vi "断电保存变量.vi"() -> ()   [LabVIEW 2016, in "斯坦道多参数.lvlib"]
panel:
  in  "盐度自动获取":bool=TRUE
  out "大气压补偿":dbl=101.35
  out "盐度补偿":dbl
  in  "浊度标液2":dbl
  in  "浊度标液1":dbl
  in  "DO标液2":dbl
  in  "DO标液1":dbl
  in  "叶绿素a标液2":dbl
  in  "叶绿素a标液1":dbl
  in  "pH温度偏移补偿":dbl
  in  "Turb温度偏移补偿":dbl
  in  "Cond温度偏移补偿":dbl
  in  "DO温度偏移补偿":dbl
  in  "水样测定时间":dbl=1.0
  in  "叶绿素a启用":bool
  in  "标样核查配置":T1={"数据保存间隔"=1.0, "水温标样值"=0.0, "pH标样值"=0.0, "溶解氧标样值"=0.0, "电导率标样值"=0.0, "浊度标样值"=0.0}
  in  "Temp":bool
  in  "Cond":bool
  in  "Turb":bool
  in  "DO":bool
  in  "pH":bool
  in  "VISA资源名称":refnum<visa-resource-name>
  in  "水温通道":enum16{"NULL", "pH", "Cond", "DO", "Turb"}(ring)
  # "请设置串口参数"
  # "请选择要启用的参数"
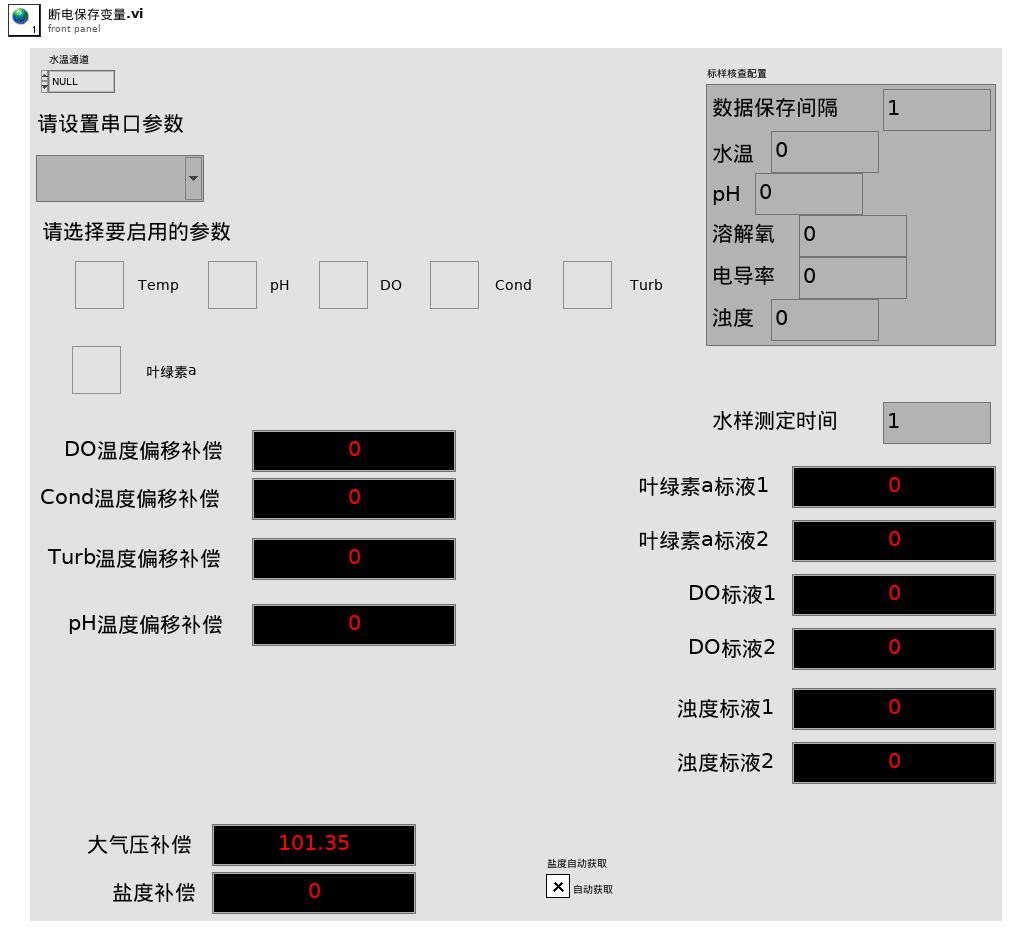
[diagram p1: front panel]
types:
  T1 = cluster{"数据保存间隔":dbl, "水温标样值":dbl, "pH标样值":dbl, "溶解氧标样值":dbl, "电导率标样值":dbl, "浊度标样值":dbl}
diagram:
